vi "3 dof forward.vi"() -> ()   [LabVIEW 2021]
panel:
  in  "Parameters of 3 DOF":T1={"Theta Motor 1"=0.0, "Theta Motor 2"=0.0, "l1"=230.59, "l2"=112.96, "l3"=112.96, "Theta Motor 3"=0.0} caption="Parameters of Delta Robot"
  out "Coordinates":cluster{"x":dbl, "y":dbl, "y 2":dbl, "y 3":dbl}
  # "Definitions about the Inputs of Forward Kinematics :"
  # "Theta Motor 1 , Theta Motor 2 and Theta Motor 3 represents the angles of thee smart motors of 2 DOF."
  # "l1 and l2 and l3 respresents links length."
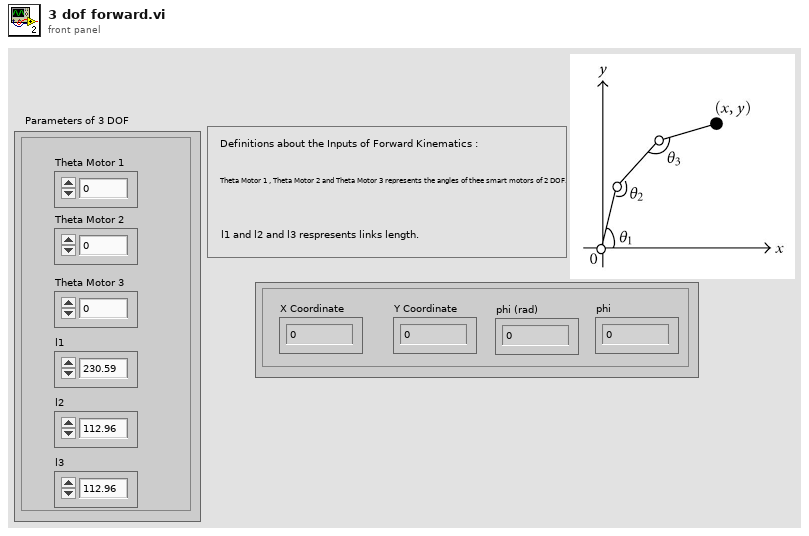
[diagram p1: front panel]
types:
  T1 = cluster{"Theta Motor 1":dbl, "Theta Motor 2":dbl, "l1":dbl, "l2":dbl, "l3":dbl, "Theta Motor 3":dbl}
  T2 = cluster{"X":dbl, "Y":dbl, "phi":dbl, "phi_dg":dbl}
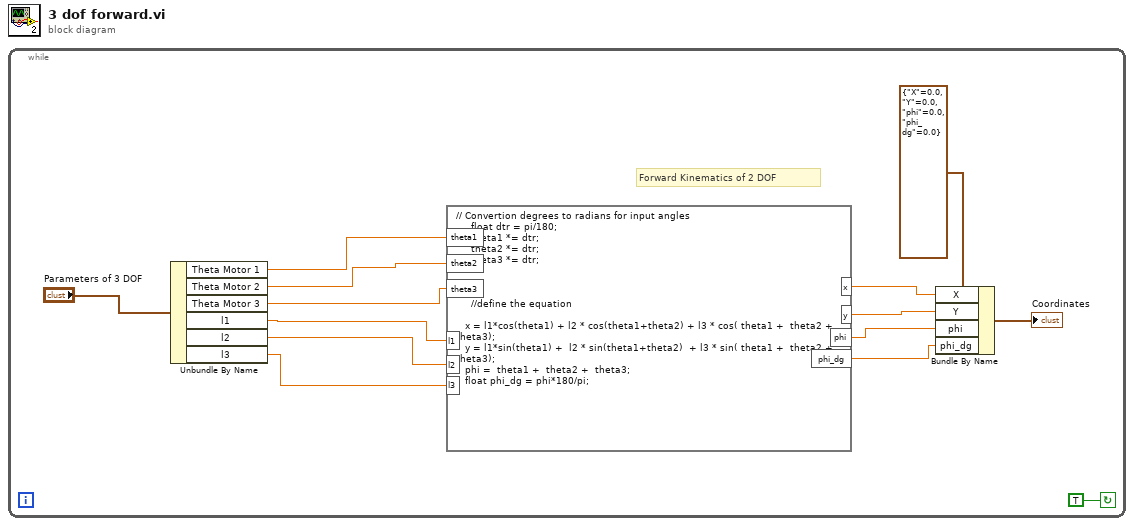
[diagram p0: block diagram]
diagram:
  n1 = while {
    stop <- TRUE continue-if-true
    # "Forward Kinematics of 2 DOF"
    n2 = Unbundle By Name "Unbundle By Name"("Parameters of 3 DOF") -> ("Theta Motor 1"=w13:dbl, "Theta Motor 2"=w6:dbl, "Theta Motor 3"=w5:dbl, "l1"=w4:dbl, "l2"=w3:dbl, "l3"=w2:dbl)
    n3 = formula code="// Convertion degrees to radians for input angles\n     float dtr = pi/180;\n     theta1 *= dtr;\n     theta2 *= dtr;\n     theta3 *= dtr;\n     \n     \n  \n     //define the equation\n\n   x = l1*cos(theta1) + l2 * cos(theta1+theta2) + l3 * cos( theta1 +  theta2 +  theta3);\n   y = l1*sin(theta1) +  l2 * sin(theta1+theta2)  + l3 * sin( theta1 +  theta2 +  theta3);\n   phi =  theta1 +  theta2 +  theta3;\n   float phi_dg = phi*180/pi;"("theta1"=w13, "theta2"=w6, "l1"=w4, "l2"=w3, "theta3"=w5, "l3"=w2) -> ("x"=w12:dbl, "y"=w10:dbl, "phi"=w7:dbl, "phi_dg"=w1:dbl)
    n4 = Bundle By Name(cluster=T2 {"X"=0.0, "Y"=0.0, "phi"=0.0, "phi_dg"=0.0}, "X"=w12, "Y"=w10, "phi"=w7, "phi_dg"=w1) -> (→"Coordinates":T2)
  }
